vi "AutoAim.vi"(6 "StartTime(ms)":u32, 11 "FirstAim":bool) -> (3 "Complete":bool)   [LabVIEW 2019]
uses:
  Implements/Shooter/TypeDefs/Hood_Homing_State.ctl
  ArgosLib/Signal Processing/TypeDefs/EdgeDetector_Type.ctl
  Global_Var-RefNum/RobotState.vi
  Global_Var-RefNum/AutoCommands.vi
  ArgosLib/ArgosLib.lvlib
panel:
  in  "PulseTime(ms)":u32=500
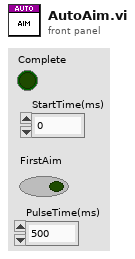
[diagram p1: front panel]
types:
  T1 = typedef "ArgosLib.lvlib/EdgeDetector_Type.ctl" = enum16{"RisingEdge", "FallingEdge", "Both"}
  T2 = typedef "Hood_Homing_State.ctl" = enum16{"Not Homed", "Homing in Process", "Homing Failed", "Homing Completed"}
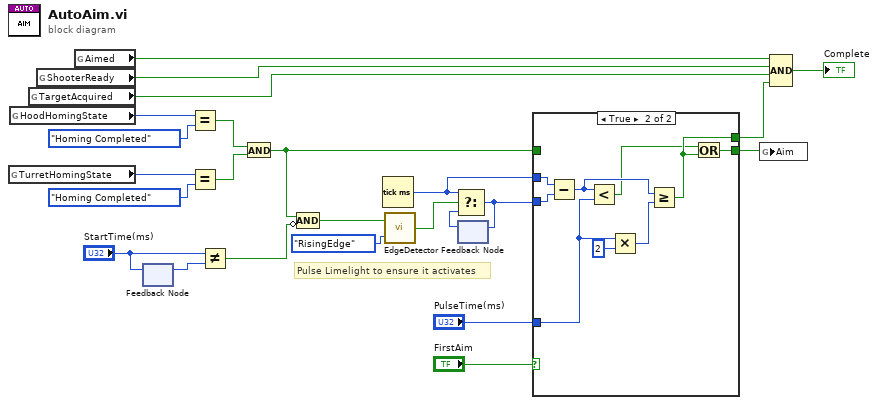
[diagram p0: block diagram]
diagram:
  # "Pulse Limelight to ensure it activates"
  n1 = global read "RobotState.vi" "TurretHomingState"() -> (w24:T2)
  n2 = global read "RobotState.vi" "HoodHomingState"() -> (w21:T2)
  n3 = global read "RobotState.vi" "TargetAcquired"() -> (w16:bool)
  n4 = global read "RobotState.vi" "ShooterReady"() -> (w17:bool)
  n5 = global read "RobotState.vi" "Aimed"() -> (w18:bool)
  n6 = feedback-in #1("StartTime(ms)") -> ()
  n7 = feedback #1() -> (w13:u32)  [unwired: 1 in]
  n8 = Equal?(x=w21, y=Hood_Homing_State."Homing Completed") -> (x = y?=w20:bool)
  n9 = Equal?(x=w24, y=Hood_Homing_State."Homing Completed") -> (x = y?=w19:bool)
  n10 = Not Equal?(x="StartTime(ms)", y=w13) -> (x != y?=w12:bool)
  n11 = And(x=w20, y=w19) -> (x .and. y?=w3:bool)
  n12 = Compound Arithmetic op=AND(w3, invert w12) -> (w11:bool)
  n13 = Tick Count (ms)() -> (millisecond timer value=w4:u32)
  n14 = call "EdgeDetector.vi"("DetectorType"=EdgeDetector_Type."RisingEdge", "Input"=w11) -> ("Edge"=w9:bool)
  n15 = feedback #2() -> (w8:u32)  [unwired: 1 in]
  n16 = Select(t=w4, s=w9, f=w8) -> (s? t:f=w5:u32)
  n17 = feedback-in #2(w5) -> ()
  n18 = case shown="True" "FirstAim" {
    tunnel: "PulseTime(ms)" -> [_ w31]
    tunnel: w5 -> [_ w33]
    tunnel: w4 -> [_ w34]
    tunnel: w3 -> [w25 _]
    tunnel: [w25 w28] -> w2
    tunnel: [w25 w27] -> w1
    frame False {
    }
    frame True {
      n19 = Subtract(x=w34, y=w33) -> (x-y=w32:u32)
      n20 = Less?(x=w32, y=w31) -> (x < y?=w26:bool)
      n21 = Multiply(x=w31, y=u32 2) -> (x*y=w29:u32)
      n22 = Greater Or Equal?(x=w32, y=w29) -> (x >= y?=w27:bool)
      n23 = Or(x=w26, y=w27) -> (x .or. y?=w28:bool)
    }
  }
  n24 = global write "AutoCommands.vi" "Aim"(w2) -> ()
  n25 = Compound Arithmetic op=AND(w18, w17, w16, w1) -> (→"Complete":bool)
